vi "Data Analysis 2017a.vi"() -> ()   [LabVIEW 2016]
uses:
  controls/measurement type.ctl
  controls/analysis control.ctl
  controls/sequence calculation technique.ctl
  <vilib>/Utility/miscctls.llb/LVRowAndColumnTypeDef.ctl
  <vilib>/addons/database/Connection.llb/DB Tools Open Connec (String).vi
  <vilib>/addons/database/Connection.llb/Conn Execute.vi
  <vilib>/addons/database/Recordset.llb/Rec Fetch Recordset Data (R).vi
  <vilib>/addons/database/Recordset.llb/Rec Destroy - Connection.vi
  <vilib>/Utility/file.llb/Write Delimited Spreadsheet (string).vi
  <vilib>/addons/database/NI_Database_API.lvlib
panel:
  in  "ss ratio":u16(ring) items=["other", "36Cl"]
  out "appended array":string[](array[string])
  out "Get cycle list error":errorcluster
  out "Workspace SQL querry":errorcluster
  out "Current wheel SQL query error":errorcluster
  out "Initial SQL query error":errorcluster
  out "Open DB connection error":errorcluster
  out "number of cycle used":string
  in  "cycle data":string(combo)="Sequence results"
  in  "sample name":i32(listbox)
  in  "wheelnumber":string(combo)="6"
  in  "runnumber":string(combo)="201324"
  in  "charge state":dbl=7.0
  in  "17 or 9":T1="slow switching"
  in  "Work Space  information":i32(listbox)
  in  "Standard information":i32(listbox)=-1
  in  "Stop":bool
  in  "current wheel Button":bool
  out "Work Space":T2(graph) caption="Standard"
  out "Sample Results":i32(listbox)=-1
  out "Standard":T2(graph)=[{"sequence  Result"=[19.4, 24.5, 34.5, 45.5, 47.5, 70.5, 89.5, 110.5, 124.0, 150.5, 169.5, 190.5, 204.0, 230.5, 249.5, 261.0, 277.0, 288.2, 307.4, 335.5, 342.5, 370.5, 394.5, 404.5, 417.0, 437.0, 464.2, 484.2, 506.5, 526.5, 546.5, 566.5, 586.5, 607.5, 627.5, 650.5, 661.0, 681.0, 708.2, 729.0, 741.0, 765.0], "sequence  Result"=[1.4519454351800678, 1.5322298503824174, 1.4924515531429052, 1.568750763009718, 1.5845626705257017, 1.5038602152409921, 1.499599660642818, 1.4653043997612023, 1.417417108574181, 1.43322290224636, 1.386005332883471, 1.4734215520193565, 1.3676649653233424, 1.3912805254104805, 1.3648960035187565, 1.3721559148234435, 1.3545254473343946, 1.4262144737414966, 1.3429658121267454, 1.4546730155306142, 1.3572422214614888, 1.326849825416527, 1.406695010161336, 1.2841919510474027, 1.2705425905499672, 1.2964944377771745, 1.223815731796389, 1.3081249420055532, 1.1816072101334754, 1.583402133427219, 1.6095986991223747, 1.5624430291893525, 1.587549562695433, 1.5236607582630868, 1.5557833202130582, 1.442343852830882, 1.6038938799855087, 1.5342173382618518, 1.5604164708343373, 1.6087839445346876, 1.4931752422998616, 1.5628545803277822]}, {"sequence  Result"=[19.4, 19.4, 19.4, 24.5, 24.5, 24.5, 34.5, 34.5, 34.5, 45.5, 45.5, 45.5, 47.5, 47.5, 47.5, 70.5, 70.5, 70.5, 89.5, 89.5, 89.5, 110.5, 110.5, 110.5, 124.0, 124.0, 124.0, 150.5, 150.5, 150.5, 169.5, 169.5, 169.5, 190.5, 190.5, 190.5, 204.0, 204.0, 204.0, 230.5, 230.5, 230.5, 249.5, 249.5, 249.5, 261.0, 261.0, 261.0, 277.0, 277.0, 277.0, 288.2, 288.2, 288.2, 307.4, 307.4, 307.4, 335.5, 335.5, 335.5, 342.5, 342.5, 342.5, 370.5, 370.5, 370.5, 394.5, 394.5, 394.5, 404.5, 404.5, 404.5, 417.0, 417.0, 417.0, 437.0, 437.0, 437.0, 464.2, 464.2, 464.2, 484.2, 484.2, 484.2, 506.5, 506.5, 506.5, 526.5, 526.5, 526.5, 546.5, 546.5, 546.5, 566.5, 566.5, 566.5, 586.5, 586.5, 586.5, 607.5, 607.5, 607.5, 627.5, 627.5, 627.5, 650.5, 650.5, 650.5, 661.0, 661.0, 661.0, 681.0, 681.0, 681.0, 708.2, 708.2, 708.2, 729.0, 729.0, 729.0, 741.0, 741.0, 741.0, 765.0, 765.0, 765.0], "sequence  Result"=[1.468383728249596, 1.4355071421105396, nan, 1.542047617321786, 1.5224120834430488, nan, 1.502206106235623, 1.4826970000501876, nan, 1.5762978297153396, 1.5612036963040963, nan, 1.5965183488806403, 1.572606992170763, nan, 1.5233640156653534, 1.4843564148166308, nan, 1.5097567778441556, 1.4894425434414802, nan, 1.4791206216665878, 1.4514881778558169, nan, 1.4292556539004966, 1.4055785632478652, nan, 1.440636521901955, 1.4258092825907651, nan, 1.4030972220503066, 1.3689134437166353, nan, 1.498618413275244, 1.448224690763469, nan, 1.378845508975058, 1.3564844216716267, nan, 1.402110258469831, 1.38045079235113, nan, 1.3826327912325727, 1.3471592158049404, nan, 1.3721559148234435, 1.3721559148234435, nan, 1.3545254473343946, 1.3545254473343946, nan, 1.4527033962229217, 1.3997255512600715, nan, 1.3465849926131388, 1.339346631640352, nan, 1.492855565194071, 1.4164904658671575, nan, 1.367497192447788, 1.3469872504751896, nan, 1.341952038923158, 1.311747611909896, nan, 1.4646315964098864, 1.3487584239127857, nan, 1.3093129967699637, 1.2590709053248417, nan, 1.2705425905499672, 1.2705425905499672, nan, 1.2964944377771745, 1.2964944377771745, nan, 1.2568469123999981, 1.1907845511927797, nan, 1.3796216062714253, 1.236628277739681, nan, 1.3035519408704328, 1.059662479396518, nan, 1.6168534437556528, 1.5499508230987853, nan, 1.622508388804228, 1.5966890094405215, nan, 1.5705374277755824, 1.5543486306031227, nan, 1.6046828305298093, 1.5704162948610567, nan, 1.5471512504727445, 1.500170266053429, nan, 1.5607383033141904, 1.550828337111926, nan, 1.462696421024058, 1.421991284637706, nan, 1.6038938799855087, 1.6038938799855087, nan, 1.5342173382618518, 1.5342173382618518, nan, 1.5754603536949459, 1.5453725879737288, nan, 1.6150559188054283, 1.602511970263947, nan, 1.4931752422998616, 1.4931752422998616, nan, 1.5628545803277822, 1.5628545803277822, nan]}]
  out "Row":i32
  out "Initialization error":errorcluster
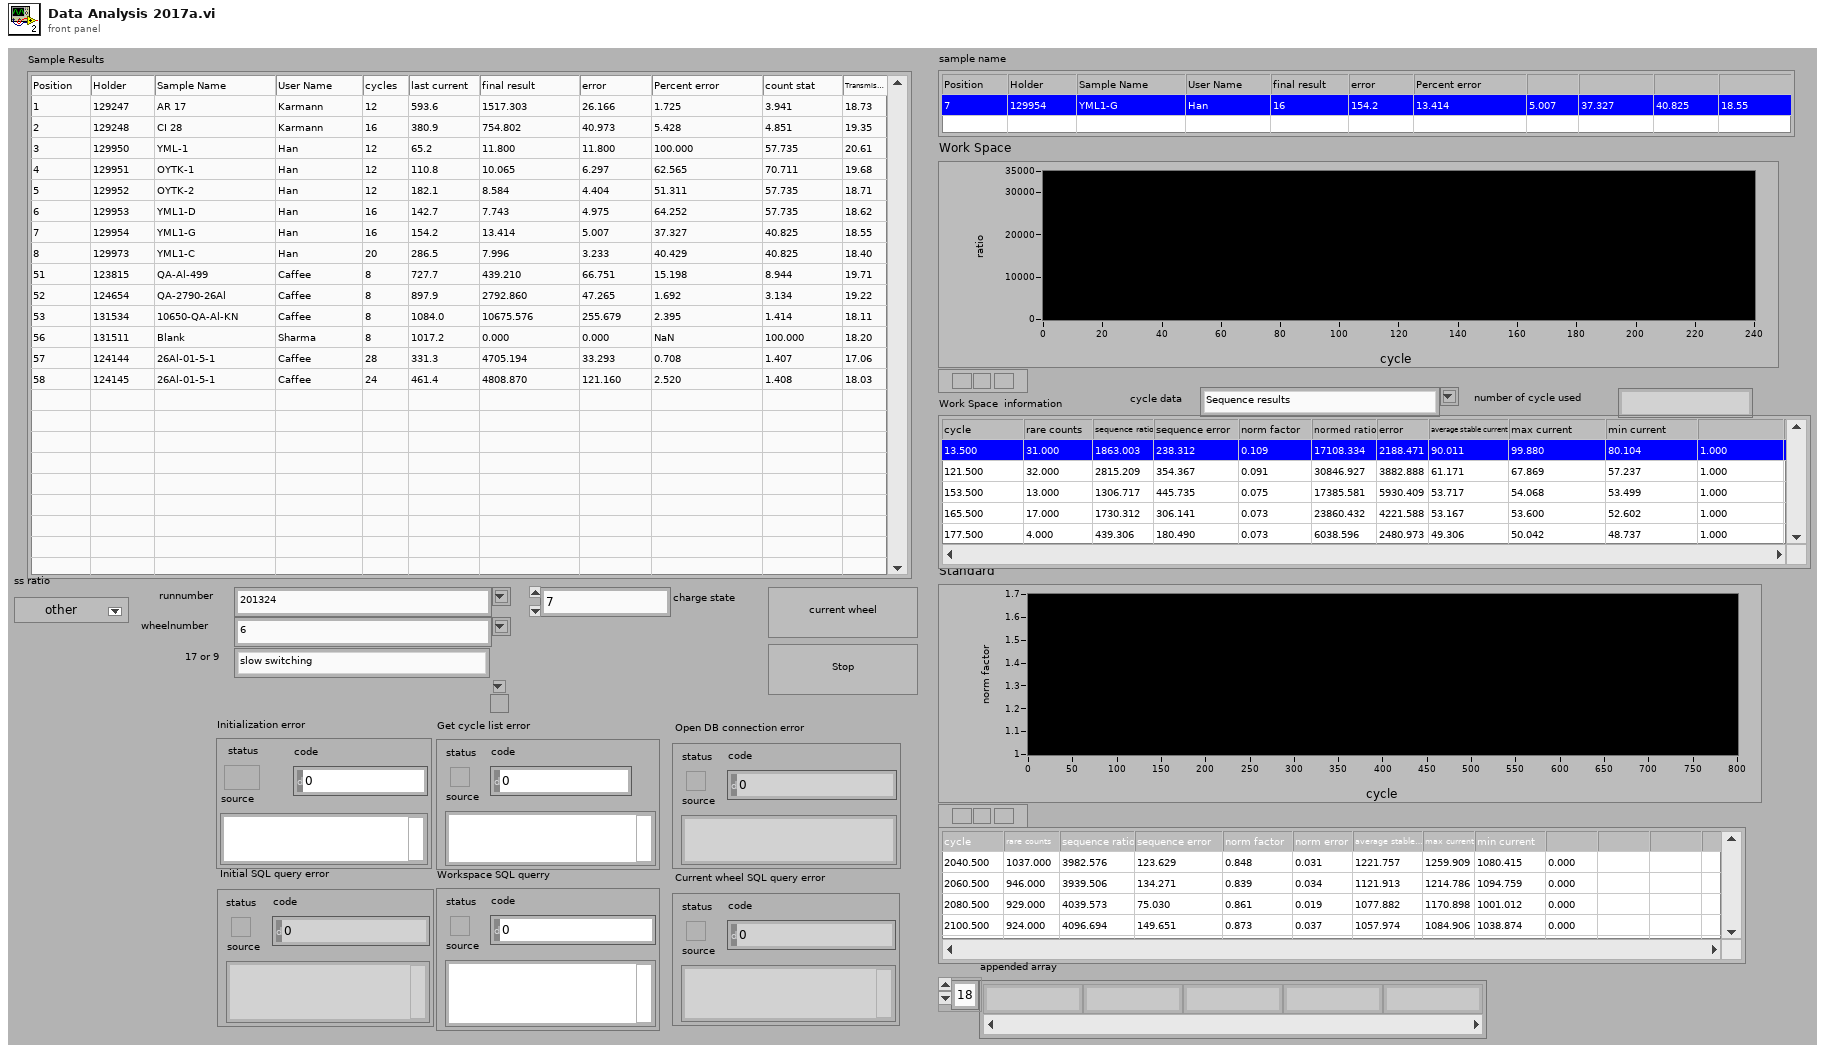
[diagram p1: front panel]
types:
  T1 = typedef "measurement type.ctl" = string
  T2 = cluster{"sequence  Result":dbl[], "sequence  Result":dbl[]}[]
  T3 = typedef "analysis control.ctl" = string
  T4 = typedef "NI_Database_API.lvlib/Conn ObjectReference.ctl" = refnum<k1>
  T5 = typedef "NI_Database_API.lvlib/Rec ObjectReference.ctl" = refnum<k1>
  T6 = typedef "sequence calculation technique.ctl" = string
  T7 = typedef "LVRowAndColumnTypeDef.ctl" = cluster{"Row":i32, "Column":i32}
  T8 = cluster{"last currents":dbl[], "number of cycles":i32[], "count stat":dbl[]}
  T9 = typedef "cycle results control.ctl" = cluster{"sample info":string[][], "cycle results labels":string[], "cycle results dbl":dbl[][]}
  T10 = typedef "data control cluster.ctl" = cluster{"Final result header":string[], "sequence result header":string[], "cycle result header ":string[], "Final Result":string[][], "sequence  Result":dbl[][], "Cycle data by seq":dbl[][][], "Cycle data by position":dbl[][][], "Final seq  Result":dbl[][], "only specific type":dbl[][]}
  T11 = typedef "LVPoint32TypeDef.ctl" = cluster{"Horizontal":i32, "Vertical":i32}
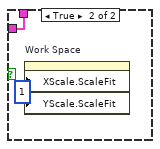
[diagram p2: hidden frame]
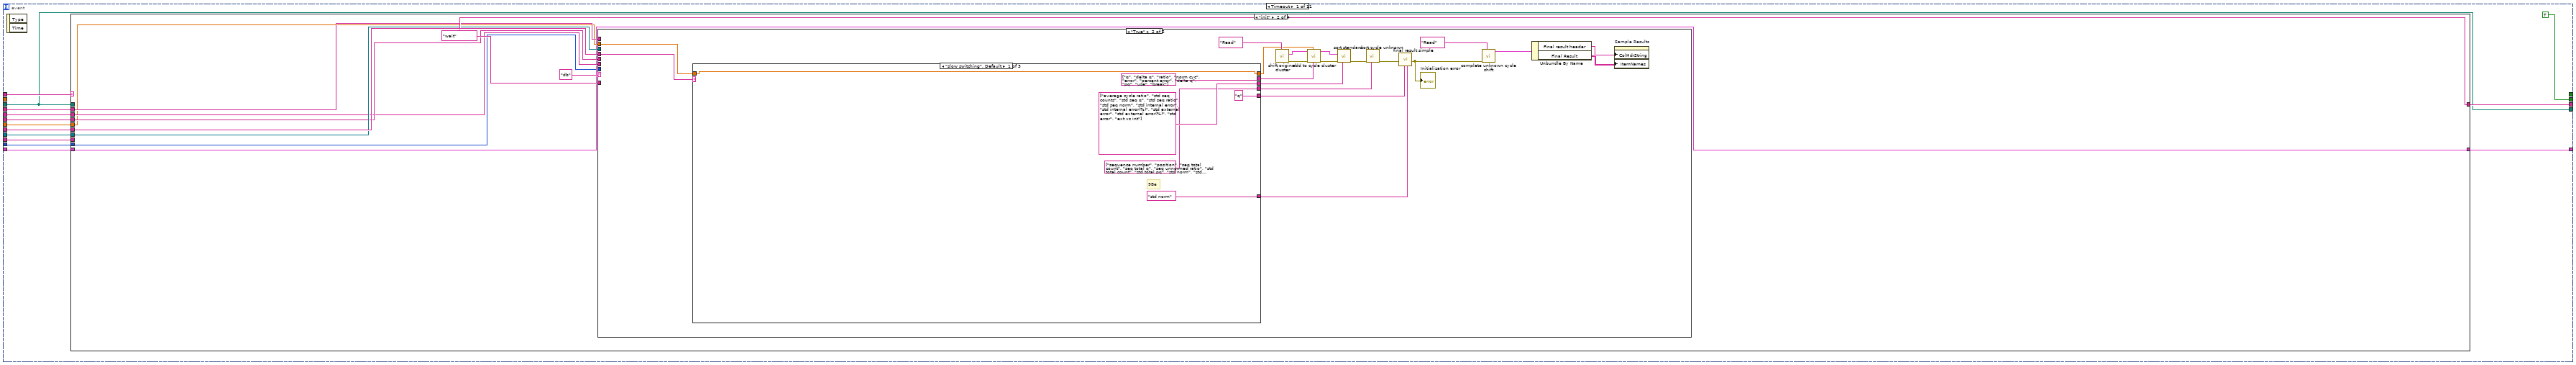
[diagram p3: hidden frame]
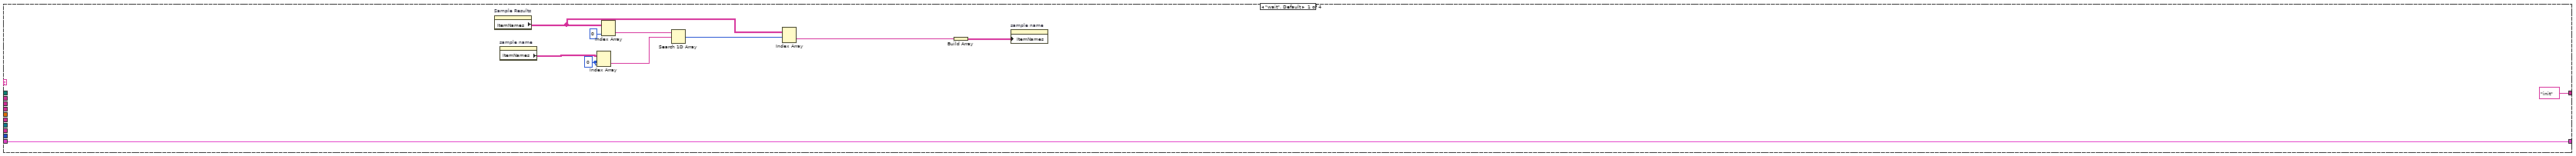
[diagram p4: hidden frame]
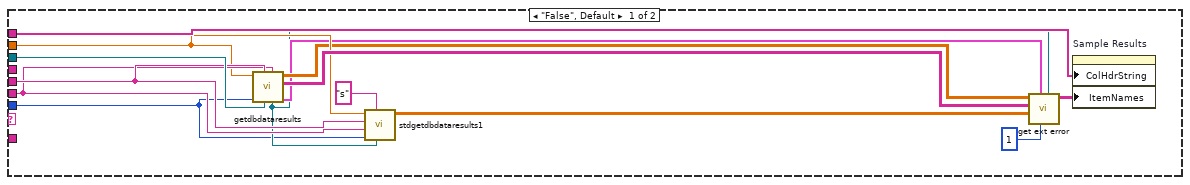
[diagram p5: hidden frame]
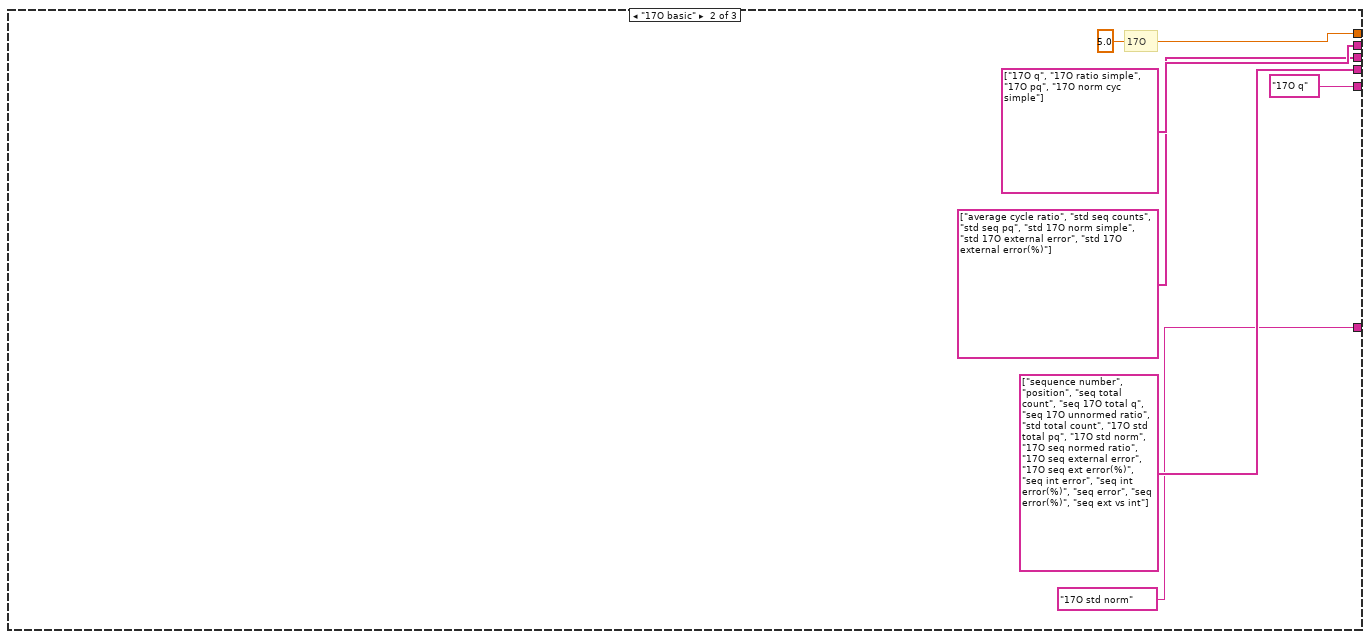
[diagram p6: hidden frame]
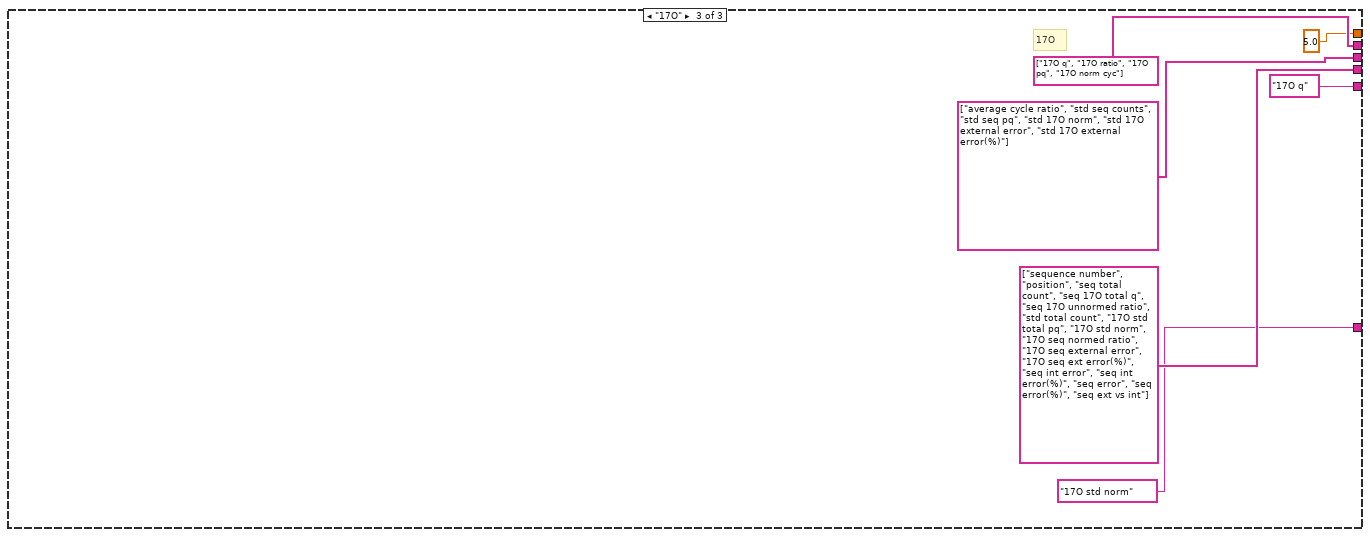
[diagram p7: hidden frame]
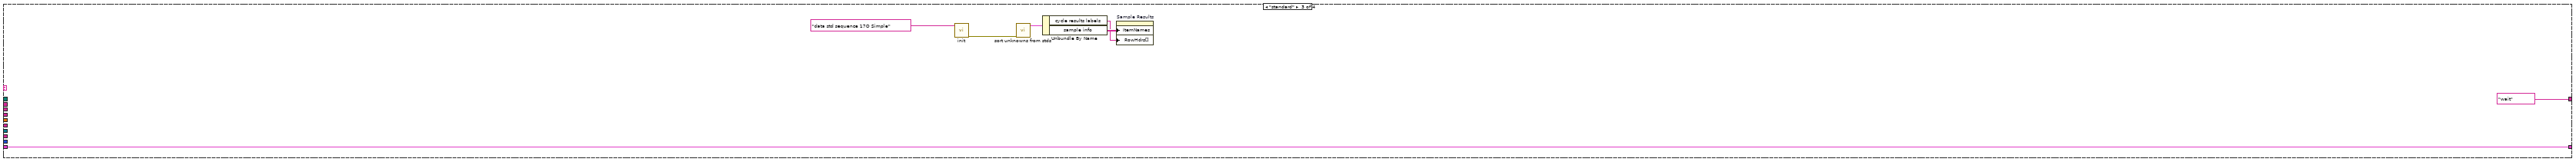
[diagram p8: hidden frame]
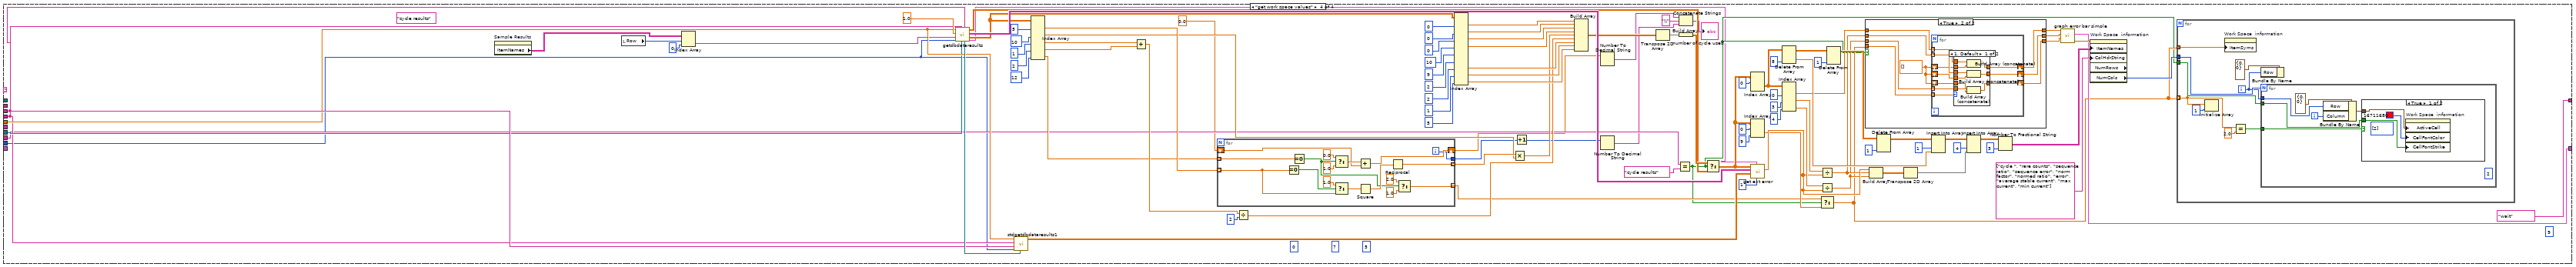
[diagram p9: hidden frame]
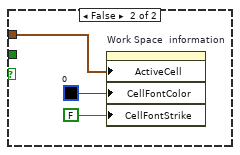
[diagram p12: hidden frame]
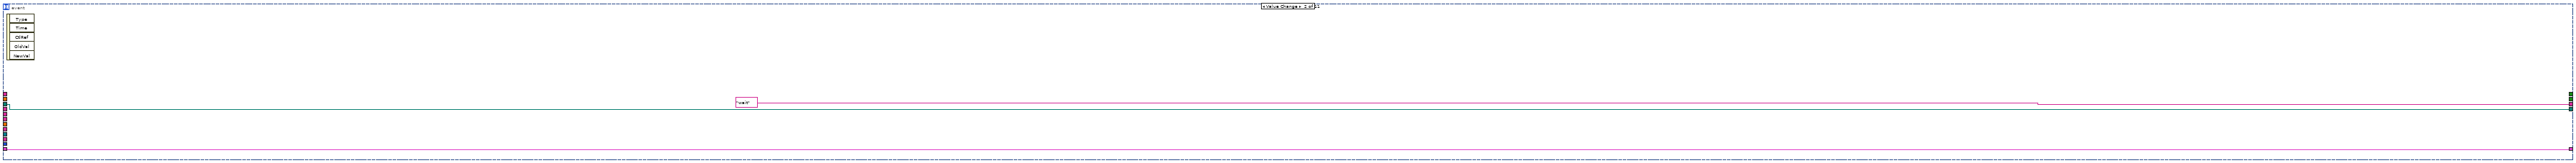
[diagram p13: hidden frame]
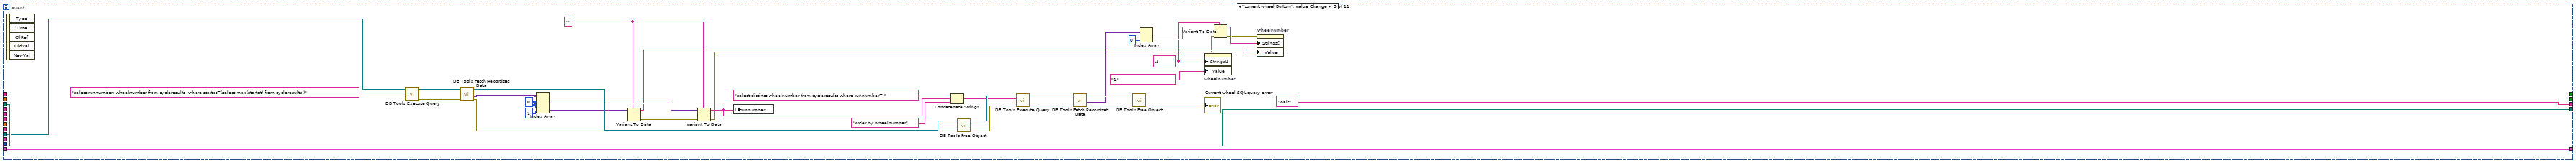
[diagram p14: hidden frame]
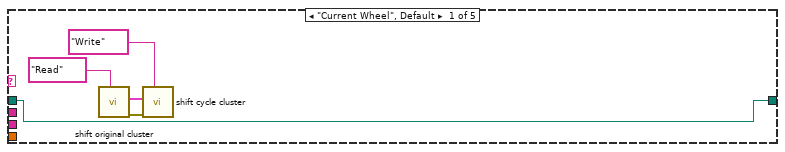
[diagram p15: hidden frame]
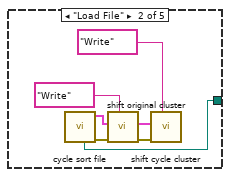
[diagram p16: hidden frame]
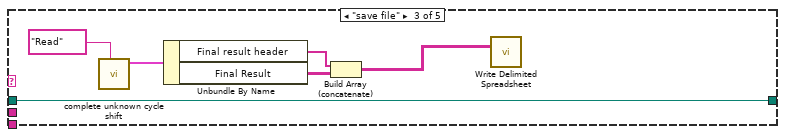
[diagram p17: hidden frame]
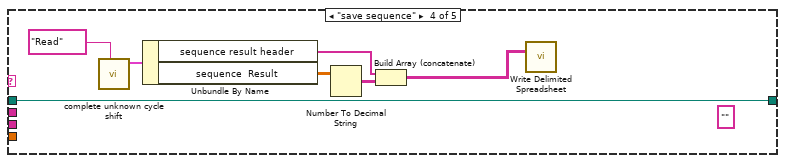
[diagram p18: hidden frame]
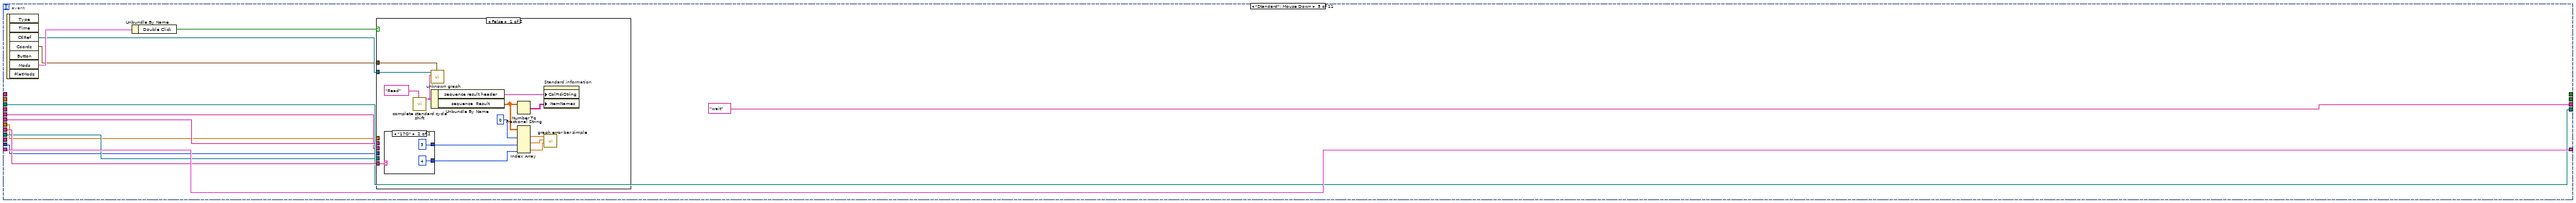
[diagram p19: hidden frame]
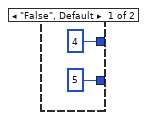
[diagram p20: hidden frame]
diagram:
  w6 = string[] [] ("Strings []")
  w33 = 0 ("disabled index (col)")
  n1 = call-poly <vilib>:"DB Tools Open Connection.vi"("connection information"="amsrecord") -> ("error out"=→"Open DB connection error":errorcluster, "connection reference"=w15:T4)  [unwired: 7 in]
  n2 = call-poly <vilib>:"DB Tools Execute Query.vi"("SQL query"="select distinct runletter, runnumber startat from cycleresults order by startat  ", "connection reference"=w15) -> ("error out"=w19:errorcluster, "recordset reference"=w21:T5)  [unwired: 6 in]
  n3 = call-poly <vilib>:"DB Tools Fetch Recordset Data.vi"("error in (no error)"=w19, "recordset reference"=w21) -> ("error out"=w18:errorcluster, "recordset data"=w22:variant[][], "recordset reference out"=w20:T5)  [unwired: 3 in]
  n4 = call-poly <vilib>:"DB Tools Free Object.vi"("error in (no error)"=w18, "recordset reference"=w20) -> ("error out"=w17:errorcluster, "connection reference"=w16:T4)  [unwired: 8 in]
  n5 = call-poly <vilib>:"DB Tools Execute Query.vi"("error in (no error)"=w17, "SQL query"="select runnumber, wheelnumber from cycleresults  where startat=(select max(startat) from cycleresults )", "connection reference"=w16) -> ("error out"=w35:errorcluster, "recordset reference"=w28:T5)  [unwired: 5 in]
  n6 = Variant To Data(type=string[][] [] ("Strings []"), Variant=w22) -> (data=w24:string[][])  [unwired: 1 in, 1 out]
  n7 = call-poly <vilib>:"DB Tools Fetch Recordset Data.vi"("error in (no error)"=w35, "recordset reference"=w28) -> ("error out"=w36:errorcluster, "recordset data"=w32:variant[][], "recordset reference out"=w29:T5)  [unwired: 3 in]
  n8 = Index Array(array=w24, index (col) #1=0 ("disabled index (col)"), index (col) #2=1 ("index (col)")) -> (element #1=w10:string[], element #2=w11:string[])  [unwired: 2 in]
  n9 = Index Array(array=w32, index (row) #1=w33, index (col) #1=w33, index (row) #2=w33, index (col) #2=1 ("disabled index (col)")) -> (element #1=w30:variant, element #2=w50:variant)
  n10 = for {
    tunnel: w10 -> [w60] mode=indexing
    tunnel: w11 -> [w59] mode=indexing
    tunnel: [w58] -> w13 mode=indexing
    n11 = Bundle(w60, w59) -> (w58:cluster{string, string})  [unwired: 1 in]
  }
  n12 = Variant To Data(type="", Variant=w30) -> (data=w1:string, error out=w4:errorcluster)  [unwired: 1 in]
  n13 = call-poly <vilib>:"DB Tools Free Object.vi"("error in (no error)"=w36, "recordset reference"=w29) -> ("error out"=w39:errorcluster, "connection reference"=w40:T4)  [unwired: 8 in]
  n14 = local write "runnumber"(w1) -> ()
  n15 = Variant To Data(error in=w4, type="", Variant=w50) -> (data=w51:string, error out=w3:errorcluster)
  n16 = Concatenate Strings("select distinct wheelnumber from cycleresults where runnumber= " ("SQL query"), w1, " order by wheelnumber" ("string")) -> (w46:string)
  n17 = property on="runnumber" class="CmbBox"("Strings And Values[]"=w13) -> (error out=w7:errorcluster)  [unwired: 2 in, 1 out]
  n18 = call-poly <vilib>:"DB Tools Execute Query.vi"("error in (no error)"=w39, "SQL query"=w46, "connection reference"=w40) -> ("error out"=w44:errorcluster, "recordset reference"=w43:T5)  [unwired: 5 in]
  n19 = call-poly <vilib>:"DB Tools Fetch Recordset Data.vi"("error in (no error)"=w44, "recordset reference"=w43) -> ("error out"=w41:errorcluster, "recordset data"=w48:variant[][], "recordset reference out"=w42:T5)  [unwired: 3 in]
  n20 = call-poly <vilib>:"DB Tools Free Object.vi"("error in (no error)"=w41, "recordset reference"=w42) -> ("error out"=→"Initial SQL query error":errorcluster)  [unwired: 8 in, 1 out]
  n21 = Index Array(array=w48, index (col)=0) -> (element=w49:variant[])  [unwired: 1 in]
  n22 = Variant To Data(error in=w3, type=w6, Variant=w49) -> (data=w37:string[], error out=w52:errorcluster)
  n23 = property on="wheelnumber" class="CmbBox"(error in=w52, "Strings[]"=w37, "Value"=w51) -> (error out=w12:errorcluster)  [unwired: 1 in, 1 out]
  n24 = property on="wheelnumber" class="CmbBox"("Strings[]"=w6, "Value"="1" ("wheelnumber")) -> ()  [unwired: 2 in, 2 out]
  n25 = while {
    shift-right: [w77] -> _
    shift-left: T3 "init" ("analysis control") -> [w78]
    shift-right: [w66] -> _
    shift-left: _ -> [w76]
    shift-right: [w73] -> _
    shift-left: _ -> [w74]
    tunnel: w15 -> [w71]
    shift-right: [w65] -> _
    shift-left: _ -> [w63]
    tunnel: w7 -> [_]
    tunnel: w12 -> [_]
    stop <- w72 stop-if-true
    (unwired) 1 ("length")
    n26 = event shown="[3] Menu Selection (User)" {
      selector: _ -> [_ _ _ _ _ _ _ _ _ _ _]
      dyn-events: _ -> [_ _ _ _ _ _ _ _ _ _ _]
      timeout: 1000 -> [_ _ _ _ _ _ _ _ _ _ _]
      tunnel: w78 -> [w96 _ _ _ _ _ _ _ _ _ _]
      tunnel: [w94 T3 "wait" ("analysis control") T3 "wait" ("analysis control") T3 "wait" ("analysis control") T3 "wait" ("analysis control") T3 "get work space values" ("analysis control") w503 T3 "get work space values" ("analysis control") T3 "get work space values" ("analysis control") _ _] -> w77
      tunnel: [w87 w351 w387 T2 [] ("graph out") w444 w486 w501 w552 w557 _ _] -> w67
      tunnel: w76 -> [w86 w351 w387 _ w444 w486 w502 w552 w557 _ _]
      tunnel: "17 or 9" -> [w95 _ _ _ w443 _ _ _ _ _ _]
      tunnel: w74 -> [w93 w350 w386 w393 w441 w488 w500 w555 w559 _ _]
      tunnel: [w93 w350 w386 w392 w441 w488 w500 w555 w559 _ _] -> w73
      tunnel: [_ _ _ _ _ _ _ _ _ _ TRUE ("Stop")] -> w72
      tunnel: w71 -> [w92 _ w381 _ w440 _ w496 _ _ w577 _]
      tunnel: "runnumber" -> [w91 _ _ w391 w439 _ w495 _ _ w575 _]
      tunnel: "wheelnumber" -> [w90 _ _ w390 w438 _ w494 _ _ _ _]
      tunnel: string[] ["Position", "Holder", "Sample Name", "User Name", "cycles", "last current", "final result", "error", "Percent error", "count stat", "Transmission"] ("Column Header Strings[]") -> [w89 _ _ _ _ _ _ _ _ _ _]
      tunnel: "charge state" -> [w88 _ _ w389 w437 _ _ _ _ _ _]
      tunnel: "charge state" -> [_ _ _ _ _ _ w493 _ _ _ _]
      tunnel: [TRUE _ _ _ _ _ _ TRUE TRUE _ _] -> w65
      tunnel: "cycle data" -> [w85 _ _ _ _ _ w491 _ _ _ _]
      tunnel: "ss ratio" -> [w83 _ _ _ w436 _ _ _ _ _ _]
      event Timeout {
        n27 = event-data() -> ()  [unwired: 1 in, 2 out]
        n28 = case shown="\"init\"" w96 {
          tunnel: [T3 "init" ("analysis control") w116 T3 "wait" ("analysis control") T3 "wait" ("analysis control")] -> w94
          tunnel: w95 -> [_ w117 _ _]
          tunnel: w93 -> [_ _ _ _]
          tunnel: w92 -> [_ w114 _ w201]
          tunnel: w91 -> [_ w113 _ w200]
          tunnel: w90 -> [_ w112 _ w203]
          tunnel: w89 -> [_ w111 _ _]
          tunnel: w88 -> [_ w110 _ w202]
          tunnel: [w106 w109 w170 w199] -> w87
          tunnel: w86 -> [w106 w109 w170 _]
          tunnel: w85 -> [_ _ _ w197]
          tunnel: w83 -> [_ w108 _ w177]
          frame "wait", Default {
            w104 = 0 ("disabled index (col)")
            n29 = property on="Sample Results" class="MCListbox (strict)"() -> ("ItemNames"=w100:string[][])  [unwired: 2 in, 2 out]
            n30 = property on="sample name" class="MCListbox (strict)"() -> ("ItemNames"=w105:string[][])  [unwired: 2 in, 2 out]
            n31 = Index Array(array=w105, index (row)=w104, index (col)=w104) -> (element=w101:string)
            n32 = Index Array(array=w100, index (col)=0 ("disabled index (col)")) -> (element=w102:string[])  [unwired: 1 in]
            n33 = Search 1D Array(1D array=w102, element=w101) -> (index of element=w99:i32)  [unwired: 1 in]
            n34 = Index Array(array=w100, index (row)=w99) -> (element=w98:string[])  [unwired: 1 in]
            n35 = Build Array(w98) -> (w97:string[][])
            n36 = property on="sample name" class="MCListbox (strict)"("ItemNames"=w97) -> ()  [unwired: 2 in, 2 out]
          }
          frame "init" {
            w116 = T3 "wait" ("analysis control")
            n37 = case shown="\"True\"" "db" {
              tunnel: w116 -> [_ _]
              tunnel: w117 -> [_ w134]
              tunnel: w114 -> [w127 _]
              tunnel: w113 -> [w126 _]
              tunnel: w112 -> [w125 _]
              tunnel: w111 -> [w124 _]
              tunnel: w110 -> [w123 w132]
              tunnel: w108 -> [w118 _]
              frame "False", Default {
                n38 = call "getdbdataresults.vi"("wheelname"=w125, "connection reference"=w127, "runletter"=w126, "ss ratio"=w118, "charge state"=w123) -> ("sample data list"=w120:T8, "sample data"=w131:string[][], "Array 2"=w122:dbl[][][], "connection reference out"=w119:T4)  [unwired: 2 in, 1 out]
                n39 = call "stdgetdbdataresults1.vi"("connection reference"=w119, "type"="s", "ss ratio"=w118, "wheelname"=w125, "runletter"=w126, "charge state"=w123) -> ("seq std"=w130:dbl[][])  [unwired: 4 in, 1 out]
                n40 = call "get ext error.vi"("connection reference"=w119, "length"=1, "sample data list"=w120, "seq std"=w130, "sample data"=w131, "unknown data in"=w122) -> ("Array out"=w128:string[][])  [unwired: 4 in, 1 out]
                n41 = property on="Sample Results" class="MCListbox (strict)"("ColHdrString"=w124, "ItemNames"=w128) -> ()  [unwired: 2 in, 2 out]
              }
              frame "True" {
                n42 = case shown="\"slow switching\", Default" w134 {
                  tunnel: [string[] ["q", "delta q", "ratio", "norm cyc", "error", "percent error", "delta q", "pq", "use", "break"] ("data requested") string[] ["17O q", "17O ratio simple", "17O pq", "17O norm cyc simple"] ("data requested") string[] ["17O q", "17O ratio", "17O pq", "17O norm cyc"] ("data requested")] -> w140
                  tunnel: [string[] ["average cycle ratio", "std seq counts", "std seq q", "std seq ratio", "std seq norm", "std internal error", "std internal error(%)", "std external error", "std external error(%)", "std error", "ext vs int"] ("which measurements") string[] ["average cycle ratio", "std seq counts", "std seq pq", "std 17O norm simple", "std 17O external error", "std 17O external error(%)"] ("cycle results labels") string[] ["average cycle ratio", "std seq counts", "std seq pq", "std 17O norm", "std 17O external error", "std 17O external error(%)"] ("cycle results labels")] -> w139
                  tunnel: [string[] ["sequence number", "position", "seq total count", "seq total q", "seq unnormed ratio", "std total count", "std total pq", "std norm", "std external error", "std internal error", "std error", "seq ratio", "seq ext error", "seq ext error(%)", "seq int error", "seq int error(%)", "seq error", "seq error(%)", "seq ext vs int"] ("Array 5") string[] ["sequence number", "position", "seq total count", "seq 17O total q", "seq 17O unnormed ratio", "std total count", "17O std total pq", "17O std norm", "17O seq normed ratio", "17O seq external error", "17O seq ext error(%)", "seq int error", "seq int error(%)", "seq error", "seq error(%)", "seq ext vs int"] ("Array 5") string[] ["sequence number", "position", "seq total count", "seq 17O total q", "seq 17O unnormed ratio", "std total count", "17O std total pq", "17O std norm", "17O seq normed ratio", "17O seq external error", "17O seq ext error(%)", "seq int error", "seq int error(%)", "seq error", "seq error(%)", "seq ext vs int"] ("Array 5")] -> w138
                  tunnel: [w152 5.0 ("charge state") 5.0 ("charge state")] -> w137
                  tunnel: ["q" ("q") "17O q" ("q") "17O q" ("q")] -> w136
                  tunnel: ["std norm" ("norm type") "17O std norm" ("norm type") "17O std norm" ("norm type")] -> w135
                  tunnel: w132 -> [w152 _ _]
                  frame "slow switching", Default {
                    # "9Be"
                  }
                  frame "17O basic" {
                    # "17O"
                  }
                  frame "17O" {
                    # "17O"
                  }
                }
                n43 = call "shift original cluster.vi"("read write shift"="Read") -> ("error out"=w142:errorcluster, "cycle results cluster out"=w133:T9)  [unwired: 9 in]
                n44 = call "add to cycle cluster.vi"("data requested"=w140, "charge state"=w137, "error in"=w142, "input cluster"=w133) -> ("error out"=w148:errorcluster, "output cluster"=w141:T9)  [unwired: 6 in]
                n45 = call "sort standard.vi"("which measurements"=w139, "error in"=w148, "cycle results cluster in"=w141) -> ("error out"=w145:errorcluster)  [unwired: 8 in]
                n46 = call "sort cycle unknown.vi"("which order"=w138, "error in"=w145) -> ("error out"=w144:errorcluster)  [unwired: 9 in]
                n47 = call "final result simple.vi"("norm type"=w135, "q"=w136, "error in"=w144) -> ("error out"=w143:errorcluster)  [unwired: 8 in]
                "Initialization error" <- w143
                n48 = call "complete unknown cycle shift.vi"("read write shift"="Read", "error in"=w143) -> ("DATA CLUSTER out"=w150:T10)  [unwired: 8 in, 1 out]
                n49 = Unbundle By Name(w150) -> ("Final result header"=w147:string[], "Final Result"=w146:string[][])
                n50 = property on="Sample Results" class="MCListbox (strict)"("ColHdrString"=w147, "ItemNames"=w146) -> ()  [unwired: 2 in, 2 out]
              }
            }
          }
          frame "standard" {
            n51 = call "init.vi"("Which Data Technique"=T6 "data std sequence 17O Simple") -> ("error out"=w172:errorcluster)  [unwired: 9 in, 1 out]
            n52 = call "sort unknowns from stds.vi"("error in"=w172) -> ("output cluster"=w173:T9)  [unwired: 9 in, 1 out]
            n53 = Unbundle By Name(w173) -> ("cycle results labels"=w171:string[], "sample info"=w174:string[][])
            n54 = property on="Sample Results" class="MCListbox (strict)"("ItemNames"=w174, "RowHdrs[]"=w171) -> ()  [unwired: 2 in, 2 out]
          }
          frame "get work space values" {
            (unwired) 9 ("f")
            (unwired) 5 ("disabled index (col)")
            (unwired) "cycle results" ("y")
            (unwired) 0 ("index (row)")
            (unwired) 7 ("charge state")
            n55 = property on="Sample Results" class="MCListbox (strict)"() -> ("ItemNames"=w249:string[][])  [unwired: 2 in, 2 out]
            n56 = local read "Row"() -> (w195:i32)
            n57 = Index Array(array=w249, index (row)=w195, index (col)=0 ("disabled index (col)")) -> (element=w198:string)
            n58 = call "getdbdataresults.vi"("wheelname"=w203, "connection reference"=w201, "runletter"=w200, "ss ratio"=w177, "holder"=w198, "number of holders to calculate"=1.0, "charge state"=w202) -> ("sample data list"=w178:T8, "data"=w209:dbl[][], "sample data"=w273:string[][], "Array 2"=w211:dbl[][][], "connection reference out"=w250:T4)
            n59 = call "stdgetdbdataresults1.vi"("connection reference"=w250, "ss ratio"=w177, "wheelname"=w203, "runletter"=w200, "charge state"=w202) -> ("seq std"=w274:dbl[][])  [unwired: 5 in, 1 out]
            n60 = Index Array(array=w209, index (col) #1=5 ("disabled index (col)"), index (col) #2=10 ("index (col)"), index (col) #3=1 ("index (col)"), index (col) #4=2 ("index (col)"), index (col) #5=12 ("index (col)")) -> (element #1=w226:dbl[], element #2=w224:dbl[], element #3=w220:dbl[], element #4=w219:dbl[], element #5=w205:dbl[])  [unwired: 5 in]
            n61 = Add(x=w220, y=w219) -> (x+y=w218:dbl[])
            n62 = for {
              tunnel: w226 -> [w347] mode=indexing
              tunnel: [w344] -> w225 mode=indexing
              tunnel: w205 -> [w343] mode=indexing
              tunnel: [w340] -> w204 mode=indexing
              shift-right: [w335] -> w185
              shift-left: 0.0 -> [w334]
              tunnel: [w333] -> w180
              i -> [w333]
              n63 = Equal To 0?(x=w347) -> (x = 0?=w349:bool)
              n64 = Equal To 0?(x=w343) -> (x = 0?=w339:bool)
              n65 = Select(t=0.0, s=w339, f=1.0) -> (s? t:f=w336:dbl)
              n66 = Select(t=1.0, s=w349, f=w347) -> (s? t:f=w346:dbl)
              n67 = Add(x=w336, y=w334) -> (x+y=w335:dbl)
              n68 = Square(x=w346) -> (x^2=w345:dbl)
              n69 = Reciprocal(x=w345) -> (1/x=w344:dbl)
              n70 = Select(t=2.0, s=w339, f=1.0) -> (s? t:f=w340:dbl)
            }
            n71 = Divide(x=w218, y=2) -> (x/y=w216:dbl[])
            n72 = Index Array(array=w209, index (col) #1=0 ("disabled index (col)"), index (col) #2=0 ("index (col)"), index (col) #3=0 ("index (col)"), index (col) #4=10 ("index (col)"), index (col) #5=9 ("index (col)"), index (col) #6=2 ("index (col)"), index (col) #7=2 ("index (col)"), index (col) #8=1 ("index (col)"), index (col) #9=5 ("index (col)")) -> (element #1=w238:dbl[], element #2=w237:dbl[], element #3=w236:dbl[], element #4=w235:dbl[], element #7=w234:dbl[], element #8=w233:dbl[], element #9=w232:dbl[])  [unwired: 9 in, 2 out]
            n73 = Multiply(x=w225, y=w224) -> (x*y=w223:dbl[])
            n74 = Increment(x=w180) -> (x+1=w179:i32)
            n75 = Build Array(w238, w237, w236, w235, w223, w216, w234, w233, w232) -> (w231:dbl[][])
            n76 = Number To Decimal String(number=w185) -> (decimal integer string=w184:string)  [unwired: 1 in]
            n77 = Number To Decimal String(number=w179) -> (decimal integer string=w182:string)  [unwired: 1 in]
            n78 = Transpose 2D Array(2D array=w231) -> (transposed array=w230:dbl[][])
            n79 = Equal?(x=w197, y="cycle results" ("cycle data")) -> (x = y?=w187:bool)
            n80 = Concatenate Strings(w184, "\\" ("string"), w182) -> (→"number of cycle used":string)
            n81 = Build Array(w230) -> (w229:dbl[][][])
            n82 = Select(t=w229, s=w187, f=w211) -> (s? t:f=w210:dbl[][][])
            n83 = Index Array(array=w210, index (dim 0)=0 ("index (page)")) -> (element=w259:dbl[][])  [unwired: 2 in]
            n84 = Index Array(array=w210, index (dim 0)=0 ("index (page)"), index (dim 2)=9 ("disabled index (col)")) -> (element=w207:dbl[])  [unwired: 1 in]
            n85 = call "get ext error.vi"("length"=1, "sample data list"=w178, "seq std"=w274, "sample data"=w273, "unknown data in"=w210) -> ("normalized ratio"=w253:dbl[])  [unwired: 5 in, 1 out]
            n86 = Delete From Array(array=w259, index (col)=8 ("disabled index (col)")) -> (deleted portion=w269:dbl[], array with subset deleted=w265:dbl[][])  [unwired: 2 in]
            n87 = Index Array(array=w259, index (col) #1=0 ("index (page)"), index (col) #2=3 ("disabled index (col)"), index (col) #3=4 ("disabled index (col)")) -> (element #1=w194:dbl[], element #2=w254:dbl[], element #3=w255:dbl[])  [unwired: 3 in]
            n88 = Divide(x=w254, y=w253) -> (x/y=w193:dbl[])
            n89 = Divide(x=w255, y=w253) -> (x/y=w192:dbl[])
            n90 = Select(t=w204, s=w187, f=w207) -> (s? t:f=w191:dbl[])
            n91 = Delete From Array(array=w265, index (col)=1 ("disabled index (col)")) -> (array with subset deleted=w264:dbl[][])  [unwired: 2 in, 1 out]
            n92 = case shown="True" w187 {
              tunnel: w194 -> [w281 w289]
              tunnel: w193 -> [w280 w288]
              tunnel: w192 -> [w279 w287]
              tunnel: w191 -> [_ w286]
              tunnel: [w281 w284] -> w190
              tunnel: [w280 w283] -> w189
              tunnel: [w279 w282] -> w188
              frame False {
              }
              frame True {
                w285 = dbl[] []
                n93 = for {
                  tunnel: w289 -> [w298] mode=indexing
                  tunnel: w288 -> [w297] mode=indexing
                  tunnel: w287 -> [w296] mode=indexing
                  tunnel: w286 -> [w299] mode=indexing
                  shift-right: [w295] -> w284
                  shift-left: w285 -> [w290]
                  shift-right: [w294] -> w283
                  shift-left: w285 -> [w291]
                  shift-right: [w293] -> w282
                  shift-left: w285 -> [w292]
                  n94 = case shown="1, Default" w299 {
                    tunnel: w298 -> [w308 _]
                    tunnel: w297 -> [w307 _]
                    tunnel: w296 -> [w306 _]
                    tunnel: [w305 w311] -> w295
                    tunnel: [w304 w310] -> w294
                    tunnel: [w303 w309] -> w293
                    tunnel: w292 -> [w302 w309]
                    tunnel: w291 -> [w301 w310]
                    tunnel: w290 -> [w300 w311]
                    frame 1, Default {
                      n95 = Build Array (concatenate)(w308, w300) -> (w305:dbl[])
                      n96 = Build Array (concatenate)(w307, w301) -> (w304:dbl[])
                      n97 = Build Array (concatenate)(w306, w302) -> (w303:dbl[])
                    }
                    frame 2 {
                    }
                  }
                }
              }
            }
            n98 = Build Array(w253, w193, w192) -> (w252:dbl[][])
            n99 = Delete From Array(array=w264, index (col)=1 ("disabled index (col)")) -> (array with subset deleted=w263:dbl[][])  [unwired: 2 in, 1 out]
            n100 = Transpose 2D Array(2D array=w252) -> (transposed array=w251:dbl[][])
            n101 = Insert Into Array(array=w263, index (col)=1 ("disabled index (col)"), new element=w269) -> (w262:dbl[][])  [unwired: 1 in]
            n102 = Insert Into Array(array=w262, index (col)=4 ("disabled index (col)"), new element=w251) -> (w260:dbl[][])  [unwired: 1 in]
            n103 = Number To Fractional String(number=w260, precision (6)=i16 3) -> (F-format string=w276:string[][])  [unwired: 2 in]
            n104 = call "graph error bar simple.vi"("Yerror 2"=w188, "y Values"=w189, "x values"=w190) -> ("error out"=w215:errorcluster, "graph out"=w199:T2)  [unwired: 7 in]
            n105 = property on="Work Space  information" class="MCListbox (strict)" props=["ItemNames", "ColHdrString", "NumRows", "NumCols"](error in=w215, "ItemNames"=w276, "ColHdrString"=string[] ["cycle ", "rare counts", "sequence ratio", "sequence error", "norm factor", "normed ratio", "error", "average stable current", "max current", "min current"] ("Row Header Strings[]")) -> ("NumCols"=w212:u32)  [unwired: 1 in, 3 out]
            n106 = for {
              tunnel: w191 -> [w315] mode=indexing
              tunnel: w212 -> [w320]
              tunnel: w191 -> [w313]
              tunnel: w187 -> [w312]
              i -> [w316]
              n107 = Initialize Array(w315, 1 ("dimension size")) -> ()  [unwired: 1 out]
              n108 = property on="Work Space  information" class="MCListbox (strict)"("ItemSyms"=w313) -> ()  [unwired: 2 in, 2 out]
              n109 = Equal?(x=w315, y=2.0) -> (x = y?=w318:bool)
              n110 = Bundle By Name(cluster=T7 {"Row"=0, "Column"=0} ("Active Cell:Active Cell"), "Row"=w316) -> ()  [unwired: 1 out]
              n111 = for {
                N: w320 -> [_]
                tunnel: w316 -> [w325]
                tunnel: w318 -> [w322]
                tunnel: w312 -> [w321]
                i -> [w324]
                (unwired) 2
                n112 = Bundle By Name(cluster=T7 {"Row"=0, "Column"=0} ("Active Cell:Active Cell"), "Row"=w325, "Column"=w324) -> (w323:T7)
                n113 = case shown="True" w322 {
                  tunnel: w323 -> [w329 w332]
                  tunnel: w321 -> [w327 _]
                  frame True {
                    (unwired) i32[] [2] ("Item Symbols")
                    n114 = property on="Work Space  information" class="MCListbox (strict)"("ActiveCell"=w329, "CellFontColor"=u32 16711680, "CellFontStrike"=w327) -> ()  [unwired: 2 in, 2 out]
                  }
                  frame False {
                    n115 = property on="Work Space  information" class="MCListbox (strict)"("ActiveCell"=w332, "CellFontColor"=u32 0, "CellFontStrike"=FALSE ("Active Cell:Cell Font:Strikeout")) -> ()  [unwired: 2 in, 2 out]
                  }
                }
              }
            }
          }
        }
      }
      event Value Change {
        n116 = event-data() -> ()  [unwired: 1 in, 5 out]
      }
      event "current wheel Button": Value Change {
        w359 = ""
        w361 = string[] [] ("Strings []")
        w379 = 0 ("disabled index (col)")
        n117 = event-data() -> ()  [unwired: 1 in, 5 out]
        n118 = call-poly <vilib>:"DB Tools Execute Query.vi"("SQL query"="select runnumber, wheelnumber from cycleresults  where startat=(select max(startat) from cycleresults )", "connection reference"=w381) -> ("error out"=w377:errorcluster, "recordset reference"=w385:T5)  [unwired: 6 in]
        n119 = call-poly <vilib>:"DB Tools Fetch Recordset Data.vi"("error in (no error)"=w377, "recordset reference"=w385) -> ("error out"=w376:errorcluster, "recordset data"=w380:variant[][], "recordset reference out"=w384:T5)  [unwired: 3 in]
        n120 = Index Array(array=w380, index (row) #1=w379, index (col) #1=w379, index (row) #2=w379, index (col) #2=1 ("disabled index (col)")) -> (element #1=w383:variant, element #2=w360:variant)
        n121 = Variant To Data(type=w359, Variant=w360) -> (data=w358:string, error out=w357:errorcluster)  [unwired: 1 in]
        n122 = Variant To Data(error in=w357, type=w359, Variant=w383) -> (data=w366:string, error out=w356:errorcluster)
        n123 = local write "runnumber"(w366) -> ()
        n124 = Concatenate Strings("select distinct wheelnumber from cycleresults where runnumber= " ("SQL query"), w366, "order by wheelnumber" ("string")) -> (w365:string)
        n125 = call-poly <vilib>:"DB Tools Free Object.vi"("error in (no error)"=w376, "recordset reference"=w384) -> ("error out"=w373:errorcluster, "connection reference"=w372:T4)  [unwired: 8 in]
        n126 = call-poly <vilib>:"DB Tools Execute Query.vi"("error in (no error)"=w373, "SQL query"=w365, "connection reference"=w372) -> ("error out"=w368:errorcluster, "recordset reference"=w369:T5)  [unwired: 5 in]
        n127 = call-poly <vilib>:"DB Tools Fetch Recordset Data.vi"("error in (no error)"=w368, "recordset reference"=w369) -> ("error out"=w371:errorcluster, "recordset data"=w363:variant[][], "recordset reference out"=w370:T5)  [unwired: 3 in]
        n128 = call-poly <vilib>:"DB Tools Free Object.vi"("error in (no error)"=w371, "recordset reference"=w370) -> ("error out"=→"Current wheel SQL query error":errorcluster)  [unwired: 8 in, 1 out]
        n129 = Index Array(array=w363, index (col)=0) -> (element=w362:variant[])  [unwired: 1 in]
        n130 = property on="wheelnumber" class="CmbBox"("Strings[]"=w361, "Value"="1" ("wheelnumber")) -> ()  [unwired: 2 in, 2 out]
        n131 = Variant To Data(error in=w356, type=w361, Variant=w362) -> (data=w375:string[], error out=w355:errorcluster)
        n132 = property on="wheelnumber" class="CmbBox"(error in=w355, "Strings[]"=w375, "Value"=w358) -> ()  [unwired: 1 in, 2 out]
      }
      event Menu Selection (User) {
        n133 = event-data() -> ("ItemTag"=w396:string)  [unwired: 1 in, 5 out]
        n134 = case shown="\"get cycle list\"" w396 {
          tunnel: [w397 w402 w410 w420 w435] -> w392
          tunnel: w393 -> [w397 _ w410 w420 w435]
          tunnel: w391 -> [_ _ _ _ w434]
          tunnel: w390 -> [_ _ _ _ w433]
          tunnel: w389 -> [_ _ _ _ w426]
          frame "Current Wheel", Default {
            n135 = call "shift original cluster.vi"("read write shift"="Read") -> ("error out"=w400:errorcluster, "cycle results cluster out"=w398:T9)  [unwired: 9 in]
            n136 = call "shift cycle cluster.vi"("read write shift"="Write", "error in"=w400, "cycle results cluster In"=w398) -> ()  [unwired: 7 in, 2 out]
          }
          frame "Load File" {
            n137 = call "cycle sort file.vi"() -> ("error out"=w406:errorcluster, "cycle results cluster"=w404:T9, "new file path (Not A Path if cancelled)"=w402:path)  [unwired: 9 in]
            n138 = call "shift original cluster.vi"("read write shift"="Write", "error in"=w406, "cycle results cluster In"=w404) -> ("error out"=w405:errorcluster, "cycle results cluster out"=w403:T9)  [unwired: 7 in]
            n139 = call "shift cycle cluster.vi"("read write shift"="Write", "error in"=w405, "cycle results cluster In"=w403) -> ()  [unwired: 7 in, 2 out]
          }
          frame "save file" {
            n140 = call "complete unknown cycle shift.vi"("read write shift"="Read") -> ("DATA CLUSTER out"=w413:T10)  [unwired: 9 in, 1 out]
            n141 = Unbundle By Name(w413) -> ("Final result header"=w411:string[], "Final Result"=w412:string[][])
            n142 = Build Array (concatenate)(w411, w412) -> (w409:string[][])
            n143 = call-poly <vilib>:"Write Delimited Spreadsheet.vi"("2D data"=w409) -> ()  [unwired: 13 in, 2 out]
          }
          frame "save sequence" {
            (unwired) "" ("format string")
            n144 = call "complete unknown cycle shift.vi"("read write shift"="Read") -> ("DATA CLUSTER out"=w418:T10)  [unwired: 9 in, 1 out]
            n145 = Unbundle By Name(w418) -> ("sequence result header"=w421:string[], "sequence  Result"=w417:dbl[][])
            n146 = Number To Decimal String(number=w417) -> (decimal integer string=w416:string[][])  [unwired: 1 in]
            n147 = Build Array (concatenate)(w421, w416) -> (w415:string[][])
            n148 = call-poly <vilib>:"Write Delimited Spreadsheet.vi"("2D data"=w415) -> ()  [unwired: 13 in, 2 out]
          }
          frame "get cycle list" {
            n149 = Number To Decimal String(number=w426, width (-)=i16 1) -> (decimal integer string=w422:string)
            n150 = call "get list with seq.vi"("charge state"=w422, "wheelnumber"=w433, "runletter"=w434) -> ("Array"=w429:string[][])  [unwired: 8 in]
            n151 = Build Array (concatenate)(string[] ["postition", "holder number", "sample name", "user", "estimated ratio", "sample type", "start time", "cycle", "transmission", "rare counts", "live time", "rare runtime", "first current", "second current", "interference", "injector ss", "he ss", "wheel number", "wheel name", "cycle ratio", "runnumber", "sequence number", "sequence number 1", "sequence ratio", "sequence stdev", "percent stdev"] ("new element/subarray")) -> (w423:string[])
            "appended array" <- w423
            n152 = Replace Array Subset(array=w429, new element=w423, index (row)=0) -> (w427:string[][])  [unwired: 1 in]
            n153 = Array To Spreadsheet String(array=w427, 3:"" ("format string")) -> (spreadsheet string=w431:string)  [unwired: 1 in]
            n154 = Write to Text File(text=w431) -> (error out=→"Get cycle list error":errorcluster)  [unwired: 3 in, 2 out]
          }
        }
      }
      event "Standard": Mouse Down {
        n155 = event-data() -> ("CtlRef"=w446:refnum<vi>, "Coords"=w445:T11, "Mods"=w448:cluster{"Double Click":bool, "Menu Key":bool})  [unwired: 1 in, 4 out]
        n156 = Unbundle By Name(w448) -> ("Double Click"=w447:bool)
        n157 = case shown="False" w447 {
          tunnel: w446 -> [w461 _]
          tunnel: w445 -> [w462 _]
          tunnel: w443 -> [w451 _]
          tunnel: w440 -> [_ w472]
          tunnel: w439 -> [_ w471]
          tunnel: w438 -> [_ w470]
          tunnel: w437 -> [_ w469]
          tunnel: w436 -> [_ w467]
          frame False {
            n158 = case shown="\"17O\"" w451 {
              tunnel: [4 ("index (col)") 3 ("index (col)")] -> w449
              tunnel: [5 ("index (col)") 4 ("index (col)")] -> w450
              frame "False", Default {
              }
              frame "17O" {
              }
            }
            n159 = call "complete standard cycle shift.vi"("read write shift"="Read") -> ("DATA CLUSTER out"=w457:T10)  [unwired: 9 in, 1 out]
            n160 = call "unknown graph.vi"("Coords"=w462, "DATA CLUSTER in"=w457, "CtlRef"=w461) -> ()  [unwired: 7 in, 2 out]
            n161 = Unbundle By Name(w457) -> ("sequence result header"=w460:string[], "sequence  Result"=w456:dbl[][])
            n162 = Index Array(array=w456, index (col) #1=0 ("disabled index (col)"), index (col) #2=w449, index (col) #3=w450) -> (element #1=w454:dbl[], element #2=w453:dbl[], element #3=w452:dbl[])  [unwired: 3 in]
            n163 = Number To Fractional String(number=w456) -> (F-format string=w459:string[][])  [unwired: 3 in]
            n164 = property on="Standard information" class="MCListbox (strict)"("ColHdrString"=w460, "ItemNames"=w459) -> ()  [unwired: 2 in, 2 out]
            n165 = call "graph error bar simple.vi"("Yerror 2"=w452, "y Values"=w453, "x values"=w454) -> ()  [unwired: 7 in, 2 out]
          }
          frame True {
            n166 = call "stdgetdbdataresults1.vi"("connection reference"=w472, "type"="s", "ss ratio"=w467, "wheelname"=w470, "runletter"=w471, "charge state"=w469) -> ("seq std"=w476:dbl[][])  [unwired: 4 in, 1 out]
            n167 = Delete From Array(array=w476, index (col)=2 ("disabled index (col)")) -> (array with subset deleted=w474:dbl[][])  [unwired: 2 in, 1 out]
            n168 = Index Array(array=w476, index (col) #1=0 ("disabled index (col)"), index (col) #2=5 ("disabled index (col)"), index (col) #3=6 ("index (col)")) -> (element #1=w481:dbl[], element #2=w480:dbl[], element #3=w479:dbl[])  [unwired: 3 in]
            n169 = call "graph error bar simple.vi"("Yerror 2"=w479, "y Values"=w480, "x values"=w481) -> ("graph out"=→"Standard":T2)  [unwired: 7 in, 1 out]
            n170 = Number To Fractional String(number=w474, precision (6)=i16 3) -> (F-format string=w485:string[][])  [unwired: 2 in]
            n171 = property on="Standard information" class="MCListbox (strict)"("ItemNames"=w485, "ColHdrString"=string[] ["cycle ", "rare counts", "sequence ratio", "sequence error", "norm factor", "norm error", "average stable current", "max current", "min current"] ("Row Header Strings[]")) -> ()  [unwired: 2 in, 2 out]
          }
        }
      }
      event "Work Space": Mouse Down {
        n172 = event-data() -> ("Mods"=w489:cluster{"Double Click":bool, "Menu Key":bool})  [unwired: 1 in, 7 out]
        n173 = Unbundle By Name(w489) -> ()  [unwired: 1 out]
      }
      event "Work Space  information": Double Click {
        n174 = event-data() -> ("CtlRef"=w498:refnum<vi>, "Coords"=w504:T11, "Mods"=w505:cluster{"Double Click":bool, "Menu Key":bool}, "Row"=w499:i32)  [unwired: 1 in, 4 out]
        n175 = Unbundle By Name(w505) -> ()  [unwired: 1 out]
        n176 = property class="MCListbox (strict)"(reference=w498) -> ("ItemNames"=w497:string[][])  [unwired: 1 in, 2 out]
        n177 = Not Equal?(x=w491, y="Sequence results" ("cycle data")) -> (x != y?=w490:bool)
        n178 = case shown="True" w490 {
          tunnel: w498 -> [_ w543]
          tunnel: w504 -> [_ w534]
          tunnel: [T3 "get work space values" ("analysis control") T3 "get work space values" ("analysis control")] -> w503
          tunnel: w502 -> [w507 w546]
          tunnel: [w507 w546] -> w501
          tunnel: w499 -> [_ _]
          tunnel: w497 -> [_ w542]
          tunnel: w496 -> [_ w540]
          tunnel: w495 -> [_ w526]
          tunnel: w494 -> [_ w524]
          tunnel: w493 -> [_ _]
          frame False {
            n179 = local write "cycle data"("cycle results" ("cycle data")) -> ()
          }
          frame True {
            (unwired) 1.0 ("t")
            (unwired) 0.0 ("f")
            w516 = 0 ("index (row)")
            n180 = invoke class="MCListbox (strict)" method="Point To Row Column"(reference=w543, "Point"=w534) -> ("CellPosition"=w533:T7)  [unwired: 5 in, 6 out]
            n181 = Unbundle By Name(w533) -> ("Row"=w532:i32)
            n182 = Index Array(array=w542, index (row)=w532, index (col)=0 ("disabled index (col)")) -> (element=w522:string)
            n183 = Concatenate Strings("select use from cycleresults where wheelnumber=' " ("SQL query"), w524, "' and runnumber='" ("string"), w526, "' and cycle=" ("string"), w522) -> (w531:string)
            n184 = call-poly <vilib>:"DB Tools Execute Query.vi"("SQL query"=w531, "connection reference"=w540) -> ("error out"=w536:errorcluster, "recordset reference"=w545:T5)  [unwired: 6 in]
            n185 = call-poly <vilib>:"DB Tools Fetch Recordset Data.vi"("error in (no error)"=w536, "recordset reference"=w545) -> ("error out"=w535:errorcluster, "recordset data"=w530:variant[][], "recordset reference out"=w544:T5)  [unwired: 3 in]
            n186 = Index Array(array=w530, index (row)=w516, index (col)=w516) -> (element=w529:variant)
            n187 = call-poly <vilib>:"DB Tools Free Object.vi"("error in (no error)"=w535, "recordset reference"=w544) -> ("error out"=w517:errorcluster, "connection reference"=w521:T4)  [unwired: 8 in]
            n188 = Variant To Data(type=w516, Variant=w529) -> (data=w515:i32, error out=→"Workspace SQL querry":errorcluster)  [unwired: 1 in]
            n189 = Equal?(x=w515, y=0) -> (x = y?=w513:bool)
            n190 = Select(t="TRUE" ("string"), s=w513, f="FALSE" ("string")) -> (s? t:f=w510:string)
            n191 = Concatenate Strings("update cycleresults set use= " ("SQL query"), w510, " where runnumber='" ("string"), w526, "' and wheelnumber='" ("string"), w524, "' and cycle=" ("string"), w522) -> (w520:string)
            n192 = call-poly <vilib>:"DB Tools Execute Query.vi"("error in (no error)"=w517, "SQL query"=w520, "connection reference"=w521) -> ("error out"=w519:errorcluster, "recordset reference"=w518:T5)  [unwired: 5 in]
            n193 = call-poly <vilib>:"DB Tools Free Object.vi"("error in (no error)"=w519, "recordset reference"=w518) -> ()  [unwired: 8 in, 2 out]
          }
        }
      }
      event "Sample Results": Double Click {
        (unwired) -1 ("Sample Results 2")
        n194 = event-data() -> ("Row"=w550:i32)  [unwired: 1 in, 7 out]
        "Row" <- w550
        n195 = property on="Sample Results" class="MCListbox (strict)"() -> ("ItemNames"=w551:string[][])  [unwired: 2 in, 2 out]
        n196 = local write "cycle data"("Sequence results" ("cycle data")) -> ()
        n197 = Index Array(array=w551, index (row)=w550) -> (element=w549:string[])  [unwired: 1 in]
        n198 = Build Array(w549) -> (w548:string[][])
        n199 = property on="sample name" class="MCListbox (strict)"("ItemNames"=w548) -> ()  [unwired: 2 in, 2 out]
      }
      event "cycle data": Value Change {
        n200 = event-data() -> ()  [unwired: 1 in, 5 out]
      }
      event "runnumber": Value Change {
        w563 = string[] [] ("Strings []")
        n201 = event-data() -> ()  [unwired: 1 in, 5 out]
        n202 = call <vilib>:"Space Constant.vi"() -> ("String"=w574:string)
        n203 = Concatenate Strings("select distinct wheelnumber from \ncycleresults where runnumber=" ("SQL query"), w575, w574, "order by wheelnumber" ("string")) -> (w572:string)
        n204 = call-poly <vilib>:"DB Tools Execute Query.vi"("SQL query"=w572, "connection reference"=w577) -> ("error out"=w571:errorcluster, "recordset reference"=w570:T5)  [unwired: 6 in]
        n205 = call-poly <vilib>:"DB Tools Fetch Recordset Data.vi"("error in (no error)"=w571, "recordset reference"=w570) -> ("error out"=w569:errorcluster, "recordset data"=w567:variant[][], "recordset reference out"=w568:T5)  [unwired: 3 in]
        n206 = call-poly <vilib>:"DB Tools Free Object.vi"("error in (no error)"=w569, "recordset reference"=w568) -> ()  [unwired: 8 in, 2 out]
        n207 = Index Array(array=w567, index (col)=0 ("disabled index (col)")) -> (element=w565:variant[])  [unwired: 1 in]
        n208 = Variant To Data(type=w563, Variant=w565) -> (data=w564:string[])  [unwired: 1 in, 1 out]
        n209 = property on="wheelnumber" class="CmbBox"("Strings[]"=w563, "Value"="1" ("wheelnumber")) -> (error out=w562:errorcluster)  [unwired: 2 in, 1 out]
        n210 = property on="wheelnumber" class="CmbBox"(error in=w562, "Strings[]"=w564) -> ()  [unwired: 1 in, 2 out]
      }
      event "Stop": Value Change {
        n211 = event-data() -> ()  [unwired: 1 in, 5 out]
      }
    }
    "Work Space" <- w67
    n212 = case shown="False" w63 {
      tunnel: [w80 w82] -> w66
      tunnel: w67 -> [w80 w82]
      frame False {
      }
      frame True {
        w81 = u8 1 ("Y Scale.Scale Fit")
        n213 = property on="Work Space" class="XYGraph (strict)"("XScale.ScaleFit"=w81, "YScale.ScaleFit"=w81) -> ()  [unwired: 2 in, 2 out]
      }
    }
  }
  n214 = property on="Sample Results" class="MCListbox (strict)"("Value"=0 ("Sample Results"), "Item Names"=string[][] [], "Item Symbols"=i32[] []) -> ()  [unwired: 2 in, 2 out]
